vi "test2.vi"() -> ()   [LabVIEW 2017]
uses:
  MM-MotionSelect-CTRL.ctl
  <vilib>/picture/3D Picture Control/Object/Create Object (drawable).vi
  <vilib>/picture/3D Picture Control/Object/Add Object (reference).vi
  <vilib>/picture/3D Picture Control/NI_3D Picture Control.lvlib
panel:
  in  "endprogram":bool
  in  "Set Analog Frequency":dbl=1500.0
  out "MotionBuffer":dbl[][][](array[numeric])
  out "Euler":dbl[][][](array[numeric])
  out "hardwaresetup?":bool
  out "GetComponentCount":i32
  in  "stopcapture":bool
  out "3DRef":refnum<vi>
  in  "Data":enum32{"Motion", "Analog", "Digital"}(tab)
  out "3D Picture":refnum<vi>(3d-picture)
  out "MotionChart":dbl[][](graph)
  in  "Motion.Select":T1
  out "AnalgoChart":dbl[][](graph)=[[-3.997772336006174, -9.006775449961426, -0.985625781118869, 32.99368263781076, 85.00003043934697, 76.99819933623077], [-2.008636832237248, 1.9934996329247954, 6.003357030451293, -20.0085451640189, 85.00003043934697, 75.99810778163375], [-0.9945677518844628, 7.998016599565745, 3.9873042963445156, 31.006439376622485, 86.99996940046543, 76.99819933623077], [-2.008636832237248, 6.989257749170066, 0.985625781118869, 162.001159552485, 86.99996940046543, 76.99819933623077], [-2.008636832237248, 6.00451696664095, 2.0160527341067773, 268.0056151561443, 88.00256347283715, 76.99819933623077], [-6.006409168243422, -3.002258483320475, 2.0160527341067773, 320.00061007216624, 88.00256347283715, 78.99838244542481], [-7.995544672012348, -4.011017333716155, 0.985625781118869, 404.00927725061837, 86.99996940046543, 76.99819933623077], [-9.009613752365134, -7.998016599565745, -0.985625781118869, 408.01098628342214, 88.99990836158389, 75.99810778163375], [-9.009613752365134, 6.00451696664095, 5.017731249332424, 260.00219709053675, 86.99996940046543, 75.99810778163375], [-9.009613752365134, 12.0090339332819, 3.9873042963445156, 65.98736527562151, 86.99996940046543, 77.99829089082779], [-18.994293928146405, 1.0087588503956797, 0.0, 31.986449752003004, 86.99996940046543, 76.99819933623077], [-17.00515842437748, -12.0090339332819, -3.0016785152256467, 62.01287875324497, 88.00256347283715, 76.99819933623077], [-17.00515842437748, -17.004792049527172, -6.003357030451293, 69.9890743084253, 86.99996940046543, 76.99819933623077], [-13.007386088371307, -9.991516232490541, -5.017731249332424, 73.01077296584856, 86.99996940046543, 75.99810778163375], [-10.004181504249596, 7.998016599565745, -0.985625781118869, 50.00775165483363, 86.99996940046543, 75.99810778163375], [2.008636832237248, 28.00506713241339, 0.0, 28.01196322962646, 85.00003043934697, 75.99810778163375], [2.008636832237248, 28.989807914942507, 5.017731249332424, -31.006439376622485, 86.0026245117187, 75.99810778163375], [7.995544672012348, 34.009584099054344, 3.9873042963445156, -167.99011184647705, 88.00256347283715, 75.99810778163375], [11.993317008018522, 37.01184258237482, 6.988982811570162, -235.99194289371408, 86.99996940046543, 74.99801622703673], [14.996521592140233, 26.99630828201771, 3.0016785152256467, -287.0069274343555, 86.99996940046543, 74.99801622703673], [21.002930760383656, 25.002808649092916, 3.9873042963445156, -310.00994874537037, 86.99996940046543, 75.99810778163375], [29.993043184280467, 26.99630828201771, 3.9873042963445156, -299.0120545327668, 88.00256347283715, 75.99810778163375], [27.009339928627078, 25.002808649092916, 3.0016785152256467, -310.00994874537037, 86.99996940046543, 74.99801622703673], [25.000703096389827, 22.00055016577244, 5.017731249332424, -242.98812807351388, 86.99996940046543, 73.99792467243971], [21.002930760383656, 9.006775449961426, 3.9873042963445156, -77.01248199865233, 86.99996940046543, 74.99801622703673], [13.007386088371307, -4.011017333716155, -0.985625781118869, 12.00512709841134, 88.00256347283715, 75.99810778163375], [6.006409168243422, -12.993774715811016, -3.0016785152256467, 66.99459816142927, 88.00256347283715, 76.99819933623077], [3.003204584121711, -20.991791315376762, -6.003357030451293, 107.99169886484759, 88.00256347283715, 75.99810778163375], [-3.997772336006174, -18.998291682451967, -6.003357030451293, 205.99273640289934, 86.99996940046543, 74.99801622703673], [-10.004181504249596, -18.998291682451967, -5.017731249332424, 299.0120545327668, 88.99990836158389, 74.99801622703673], [-27.009339928627078, -14.002533566206695, -0.985625781118869, 336.98745657876185, 86.99996940046543, 74.99801622703673], [-31.00711226463325, -3.002258483320475, 0.0, 313.0044248923664, 86.99996940046543, 73.99792467243971], [-32.00168001651771, 12.993774715811016, 6.003357030451293, 302.98654105514333, 86.99996940046543, 73.99792467243971], [-29.993043184280467, 36.00308373197914, 16.97964413836597, 261.989440351725, 86.99996940046543, 74.99801622703673], [-24.006135344505367, 42.992341481149204, 16.97964413836597, 106.00445560365931, 88.00256347283715, 73.99792467243971], [-27.009339928627078, 33.000825248658664, 11.021088279783717, -58.99118009582171, 88.00256347283715, 73.99792467243971], [-24.006135344505367, 15.011292416602375, 3.9873042963445156, -133.00918594747802, 88.00256347283715, 72.99783311784269], [-13.007386088371307, 4.011017333716155, 2.0160527341067773, -159.9866937808695, 86.99996940046543, 73.99792467243971], [3.997772336006174, -1.0087588503956797, 0.0, -175.9935299120846, 88.00256347283715, 74.99801622703673], [18.994293928146405, -6.989257749170066, -2.0160527341067773, -159.9866937808695, 88.00256347283715, 74.99801622703673], [21.002930760383656, -22.00055016577244, -6.988982811570162, -126.01300076767822, 88.00256347283715, 72.99783311784269], [35.00488460063942, -31.007325615733865, -12.006714060902587, -151.0032653398814, 90.99984732270235, 72.99783311784269], [40.99179244041452, -31.99206639826298, -9.99066132679581, -253.00601191073696, 88.99990836158389, 73.99792467243971], [39.0026569366456, -28.989807914942507, -6.988982811570162, -144.0070801600816, 88.00256347283715, 72.99783311784269], [31.00711226463325, -28.00506713241339, -6.988982811570162, -68.00183104723702, 88.00256347283715, 73.99792467243971], [20.00836300849919, -23.994049798697237, -5.017731249332424, -64.00012201443324, 88.00256347283715, 73.99792467243971], [17.999726176261944, -20.007050532847646, 0.985625781118869, -29.999206490814732, 88.00256347283715, 73.99792467243971], [25.000703096389827, 0.0, 6.988982811570162, -64.00012201443324, 88.00256347283715, 73.99792467243971], [25.000703096389827, 9.006775449961426, 9.00503554567694, -19.001312278211145, 88.00256347283715, 72.99783311784269], [15.991089344024696, 6.00451696664095, 8.019409764558072, -25.99749745801095, 88.00256347283715, 73.99792467243971]]
  in  "Analog.Select":T1
  out "DigitalChart":dbl[][](graph)
  in  "Digital.Select":T1
  in  "startcapture":bool
  in  "connect":bool
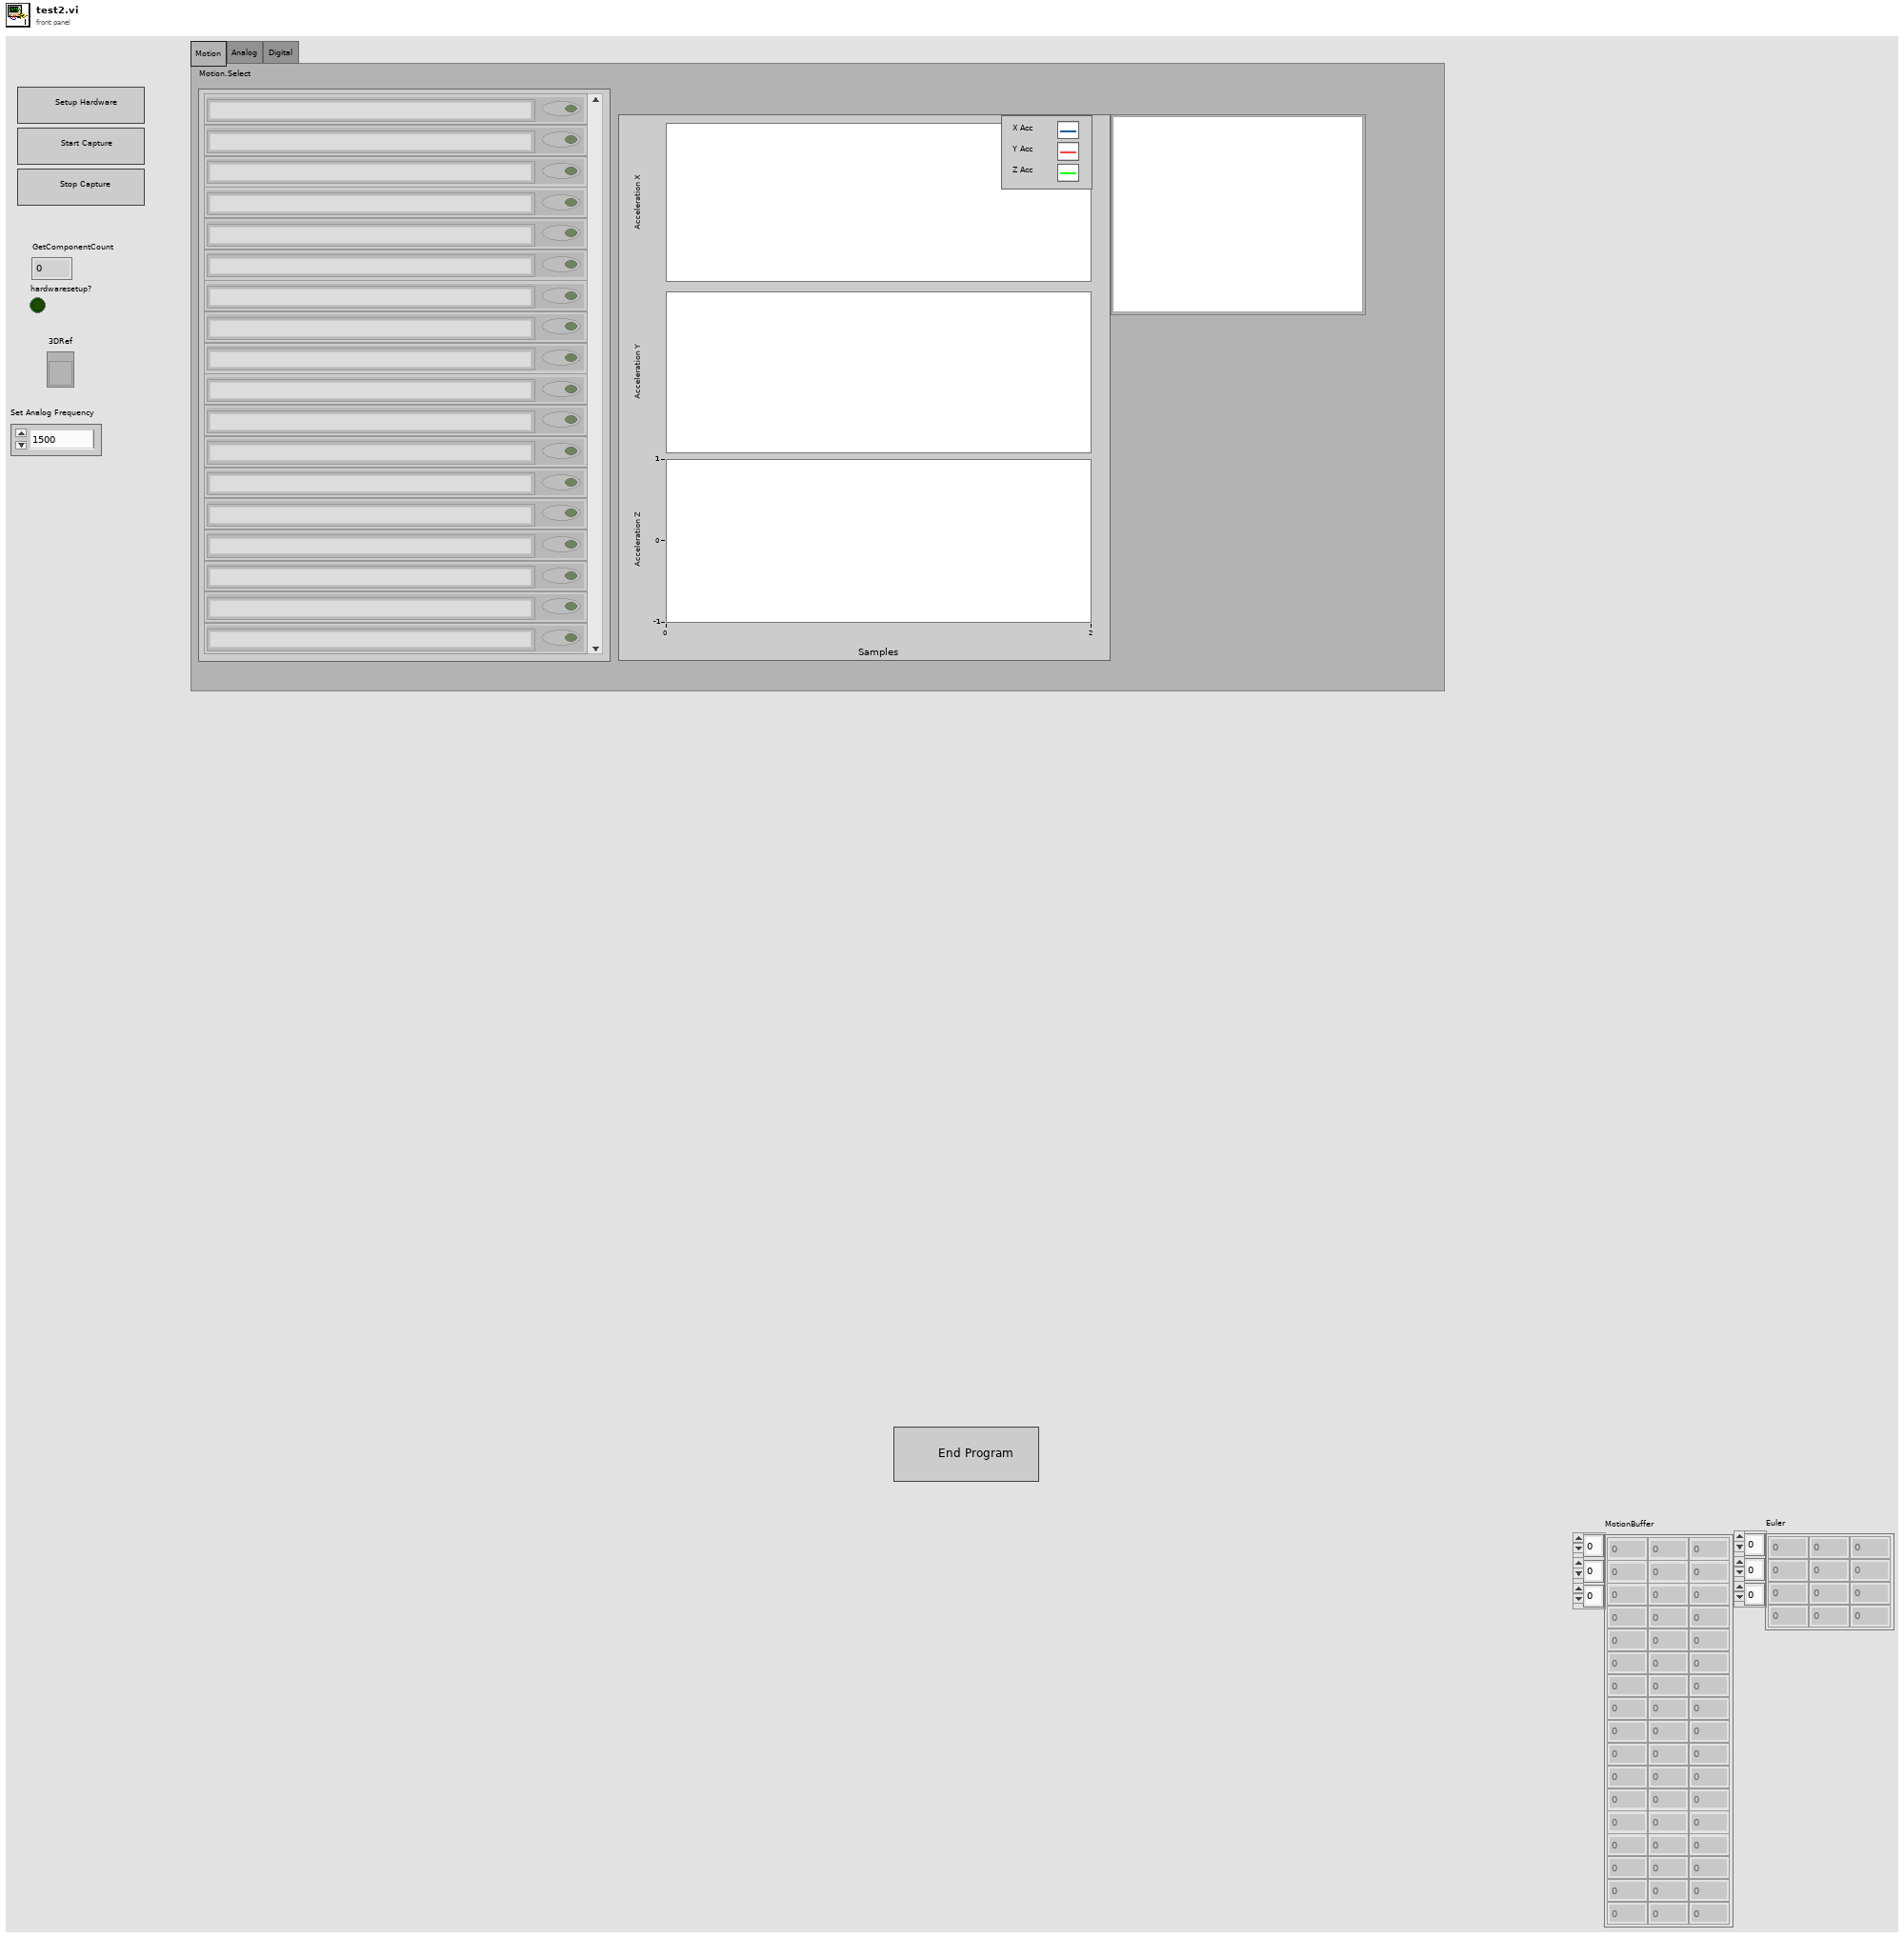
[diagram p1: front panel]
types:
  T1 = typedef "MM-MotionSelect-CTRL.ctl" = cluster{"Component":string, "Collect":bool}[]
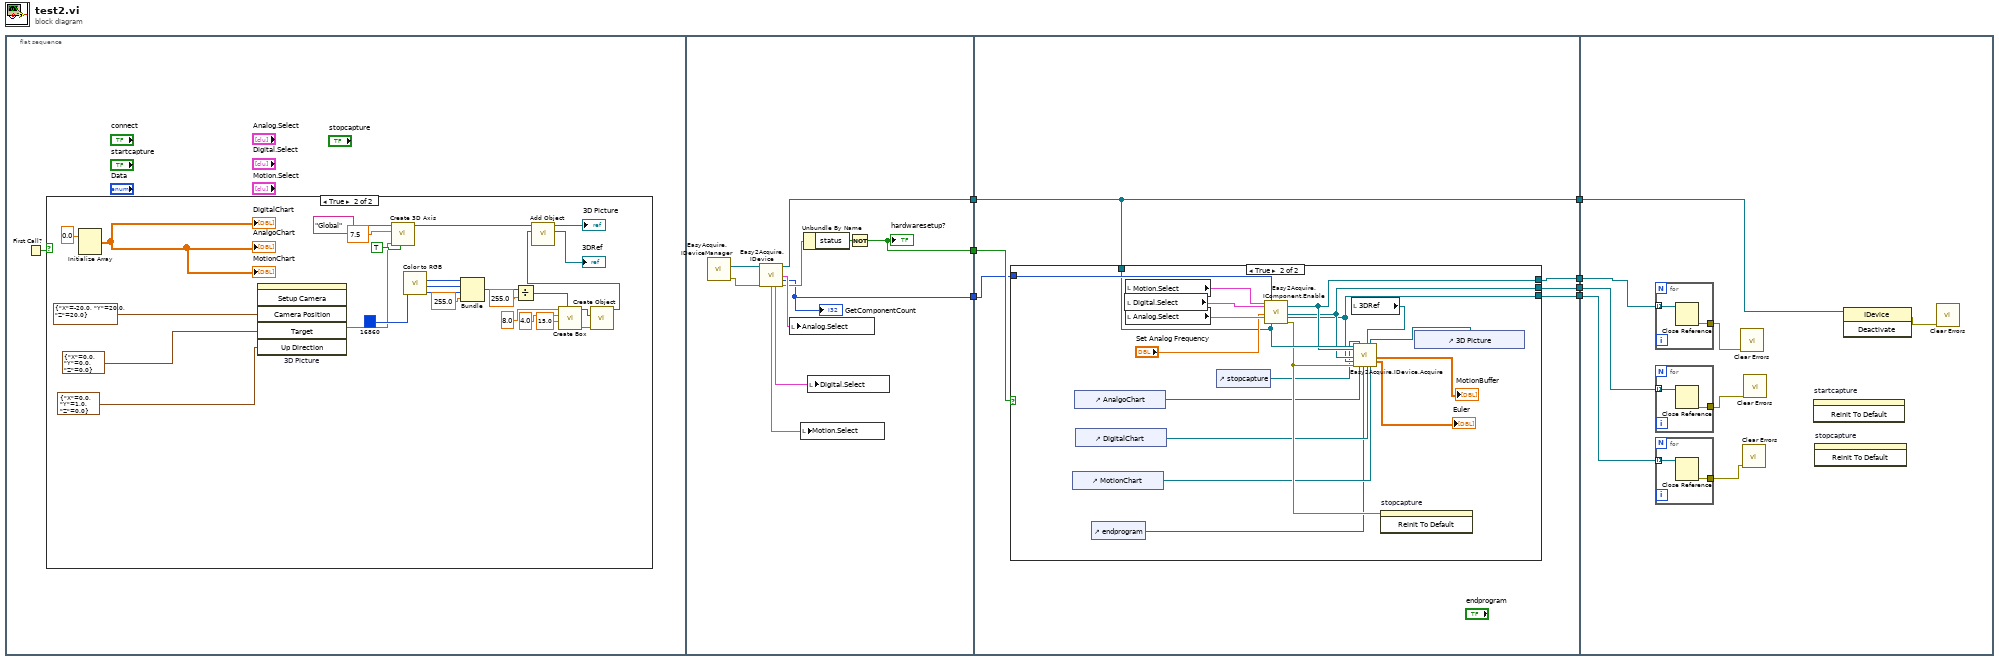
[diagram p0: block diagram]
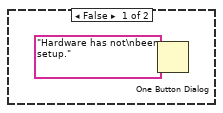
[diagram p3: hidden frame]
diagram:
  n1 = flat-sequence {
    tunnel: [w37] -> w7
    tunnel: [w36] -> w6
    tunnel: [w35] -> w5
    tunnel: w7 -> [w50]
    tunnel: w6 -> [w49]
    tunnel: w5 -> [w45]
    tunnel: [w48] -> w4
    tunnel: [w47] -> w3
    tunnel: [w46] -> w2
    tunnel: [w45] -> w1
    tunnel: w4 -> [w74]
    tunnel: w3 -> [w73]
    tunnel: w2 -> [w72]
    tunnel: w1 -> [w71]
    frame #0 {
      n2 = First Call?() -> (First Call?: T/F=w8:bool)
      n3 = case shown="True" w8 {
        frame False {
        }
        frame True {
          n4 = Initialize Array(0.0 ("element")) -> (→"DigitalChart" →"AnalgoChart" →"MotionChart":dbl[][])  [unwired: 2 in]
          n5 = invoke on="3D Picture" class="SceneGraphDisp (strict)" method="Setup Camera"("Camera Position"=cluster{"X":sgl, "Y":sgl, "Z":sgl} {"X"=-20.0, "Y"=20.0, "Z"=20.0}, "Target"=cluster{"X":sgl, "Y":sgl, "Z":sgl} {"X"=0.0, "Y"=0.0, "Z"=0.0}, "Up Direction"=cluster{"X":sgl, "Y":sgl, "Z":sgl} {"X"=0.0, "Y"=1.0, "Z"=0.0}) -> (error out=w14:errorcluster)  [unwired: 3 in, 5 out]
          n6 = call <vilib>:"Create 3D Axis.vi"("Axis label?"=TRUE, "error in (no error)"=w14, "Length"=sgl 7.5 ("Character Size"), "Name"="Global") -> ("New Object Refnum"=w18:refnum<vi>)  [unwired: 6 in, 1 out]
          n7 = call <vilib>:"Color to RGB.vi"("Color"=u32 16860 ("Color Box")) -> ("R"=w24:u8, "G"=w25:u8, "B"=w26:u8)  [unwired: 1 out]
          n8 = Bundle("R"=w24, "G"=w25, "B"=w26, 255.0) -> (w28:cluster{"R":u8, "G":u8, "B":u8, dbl})  [unwired: 1 in]
          n9 = Divide(x=w28, y=255.0) -> (x/y=w30:cluster{"R":dbl, "G":dbl, "B":dbl, dbl})
          n10 = call <vilib>:"Create Box.vi"("Color"=w30, "Length Z"=sgl 15.0, "Length Y"=sgl 4.0 ("Radius"), "Length X"=sgl 8.0 ("Height")) -> ("error out"=w21:errorcluster, "New Box Refnum"=w20:refnum<vi>)  [unwired: 6 in]
          n11 = call-poly <vilib>:"Create Object.vi"("error in (no error)"=w21, "Geometry"=w20) -> ("Scene:New Object"=w17:refnum<vi>)  [unwired: 8 in, 1 out]
          n12 = call-poly <vilib>:"Add Object.vi"("New Object In"=w17, "Scene Object In"=w18) -> ("New Object Out"=→"3DRef":refnum<vi>, "Scene Object Out"=→"3D Picture":refnum<vi>)  [unwired: 7 in, 1 out]
        }
      }
    }
    frame #1 {
      n13 = call "EasyAcquire.IDeviceManager.vi"() -> ("error out"=w40:errorcluster, "GetCurrentDevice"=w44:refnum<k7>)  [unwired: 8 in, 2 out]
      n14 = call "Easy2Acquire.IDevice.vi"("IDeviceIn"=w44, "error in"=w40) -> ("IDeviceOut"=w35:refnum<k7>, "Analog.Select"=w43:T1, "GetComponentCount"=w36:i32, "Motion.Select"=w41:T1, "Digital.Select"=w42:T1, "error out"=w39:errorcluster)  [unwired: 8 in]
      "GetComponentCount" <- w36
      n15 = local write "Analog.Select"(w43) -> ()
      n16 = local write "Motion.Select"(w41) -> ()
      n17 = Unbundle By Name(w39) -> ("status"=w38:bool)
      n18 = local write "Digital.Select"(w42) -> ()
      n19 = Not(x=w38) -> (.not. x?=w37:bool)
      "hardwaresetup?" <- w37
    }
    frame #2 {
      n20 = case shown="True" w50 {
        tunnel: w49 -> [_ w67]
        tunnel: w45 -> [_ w65]
        tunnel: [_ w64] -> w46
        tunnel: [_ w63] -> w47
        tunnel: [_ w62] -> w48
        frame False {
          n21 = One Button Dialog(message="Hardware has not\nbeen setup.") -> ()  [unwired: 1 in, 1 out]
        }
        frame True {
          n22 = control-ref of="MotionChart"() -> (w58:refnum<vi>)
          n23 = control-ref of="AnalgoChart"() -> (w55:refnum<vi>)
          n24 = control-ref of="DigitalChart"() -> (w57:refnum<vi>)
          n25 = control-ref of="endprogram"() -> (w56:refnum<vi>)
          n26 = local read "Digital.Select"() -> (w69:T1)
          n27 = local read "Motion.Select"() -> (w68:T1)
          n28 = local read "Analog.Select"() -> (w70:T1)
          n29 = control-ref of="stopcapture"() -> (w54:refnum<vi>)
          n30 = call "Easy2Acquire.IComponent.Enable.vi"("Motion.Select"=w68, "Digital.Select"=w69, "AnalogFreq"="Set Analog Frequency", "Analog.Select"=w70, "ComponentCount"=w67, "IDeviceIn"=w65) -> ("AnalogInput"=w64:refnum<k7>[], "DigitalInput"=w63:refnum<k7>[], "MotionInput"=w62:refnum<k7>[], "error out"=w61:errorcluster)  [unwired: 10 in]
          n31 = local read "3DRef"() -> (w60:refnum<vi>)
          n32 = invoke on="stopcapture" class="Bool (strict)" method="Reinit To Default"(error in=w61) -> ()  [unwired: 2 in, 3 out]
          n33 = control-ref of="3D Picture"() -> (w59:refnum<vi>)
          n34 = call "Easy2Acquire.IDevice.Acquire.vi"("IDeviceIn"=w65, "IAnalogInput"=w64, "DigitalInput"=w63, "MotionInput"=w62, "error in (no error)"=w61, "stopcapture"=w54, "AnalgoChart"=w55, "endprogram"=w56, "3DRef"=w60, "DigitalChart"=w57, "3D Picture"=w59, "MotionChart"=w58) -> ("MotionBuffer"=→"MotionBuffer":dbl[][][], "Euler"=→"Euler":dbl[][][])  [unwired: 4 in, 2 out]
        }
      }
    }
    frame #3 {
      n35 = for {
        tunnel: w72 -> [w84] mode=indexing
        tunnel: [w83] -> w78
        n36 = Close Reference(reference=w84) -> (error out=w83:errorcluster)  [unwired: 1 in]
      }
      n37 = for {
        tunnel: w73 -> [w82] mode=indexing
        tunnel: [w81] -> w77
        n38 = Close Reference(reference=w82) -> (error out=w81:errorcluster)  [unwired: 1 in]
      }
      n39 = for {
        tunnel: w74 -> [w80] mode=indexing
        tunnel: [w79] -> w76
        n40 = Close Reference(reference=w80) -> (error out=w79:errorcluster)  [unwired: 1 in]
      }
      n41 = call <vilib>:"Clear Errors.vi"("error in (no error)"=w78) -> ()  [unwired: 5 in, 2 out]
      n42 = call <vilib>:"Clear Errors.vi"("error in (no error)"=w76) -> ()  [unwired: 5 in, 2 out]
      n43 = call <vilib>:"Clear Errors.vi"("error in (no error)"=w77) -> ()  [unwired: 5 in, 2 out]
      n44 = invoke on="startcapture" class="Bool" method="Reinit To Default"() -> ()  [unwired: 3 in, 3 out]
      n45 = invoke on="stopcapture" class="Bool (strict)" method="Reinit To Default"() -> ()  [unwired: 3 in, 3 out]
      n46 = invoke class="IDevice" method="Deactivate"(reference=w71) -> (error out=w75:errorcluster)  [unwired: 2 in, 2 out]
      n47 = call <vilib>:"Clear Errors.vi"("error in (no error)"=w75) -> ()  [unwired: 5 in, 2 out]
    }
  }
